vi "ConfMappOut.vi"(8 "error in (no error)":errorcluster, 11 "ConfMapOut In":string[](array[string])) -> (0 "error out":errorcluster, 1 "Discard?":bool, 3 "ConfMapOut Out":string[](array[string]))   [LabVIEW 2014]
uses:
  TypeDefs/LogicParsedExpression.ctl
  SeqLoop.lvlib
panel:
  in  "Formula":string
  in  "Tipo de Salida":string(combo)
  in  "Stop Med":bool
  in  "Add Med":bool
  in  "Descripción":string
  in  "Nro.":i32
  in  "Nro. Hardware":i32
  in  "Bit":i32
  in  "Habilitada":bool
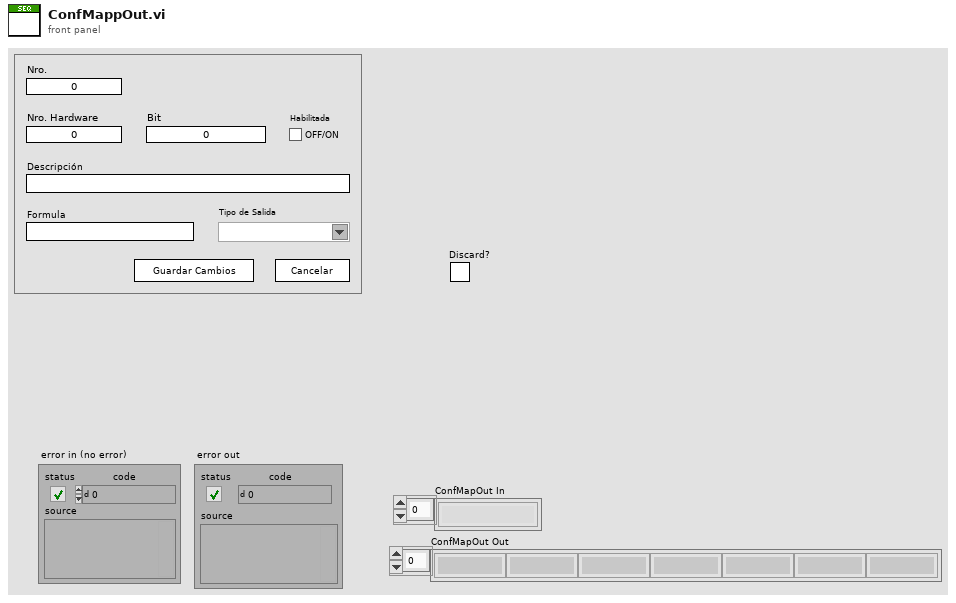
[diagram p1: front panel]
types:
  T1 = typedef "SeqLoop.lvlib/LogicParsedExpression.ctl" = cluster{"RPN ":string[], "Variables":string[], "Ctes":string[], "Formula":string, "Message":string}
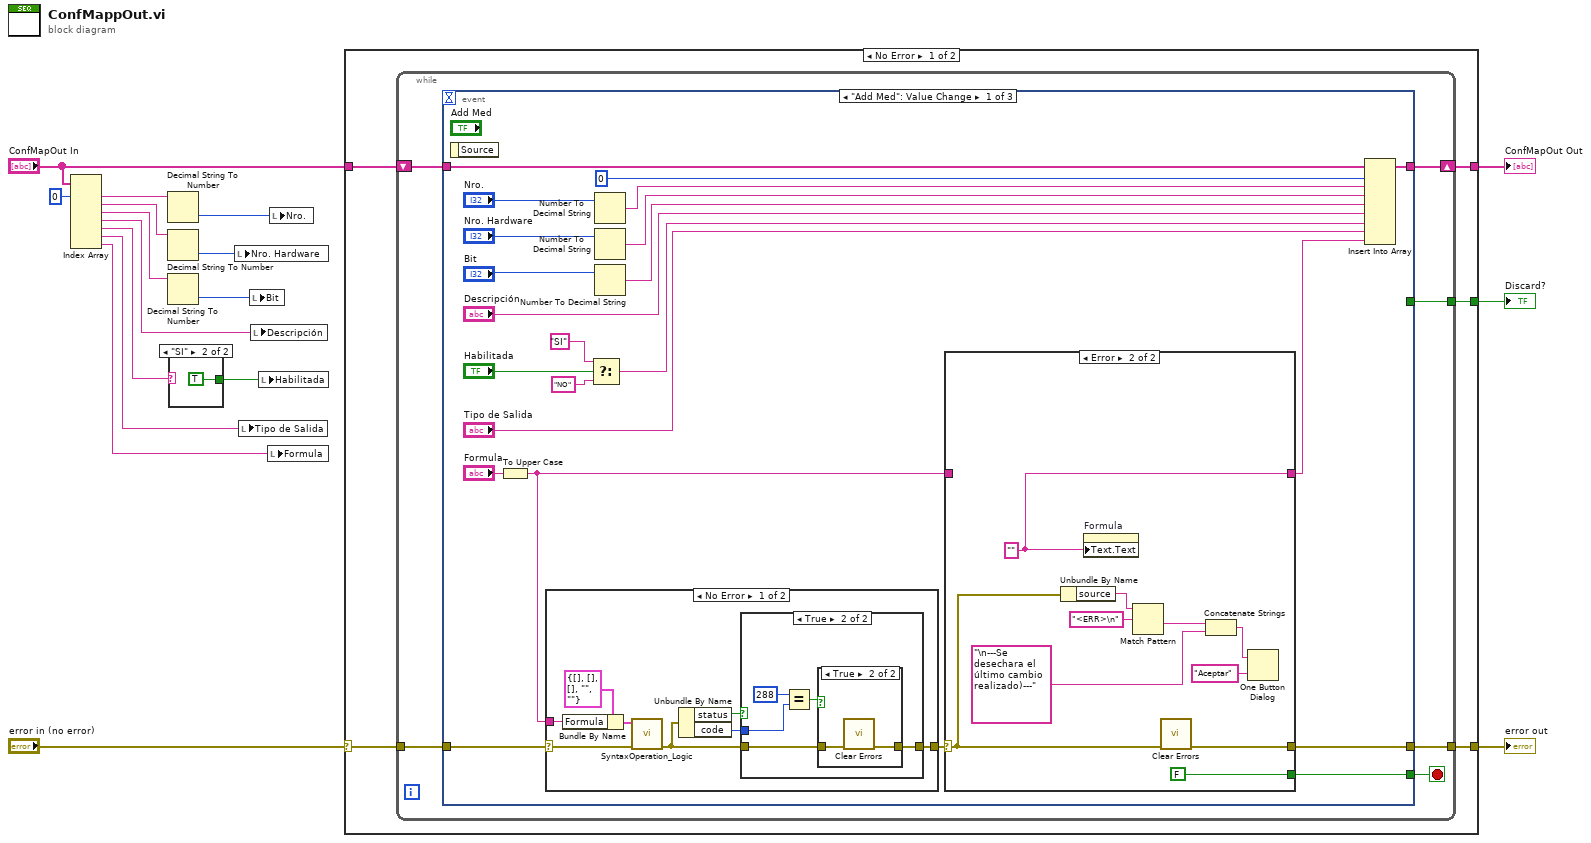
[diagram p0: block diagram]
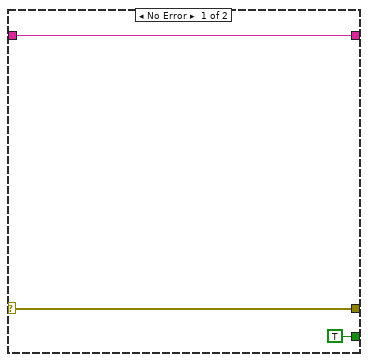
[diagram p6: hidden frame]
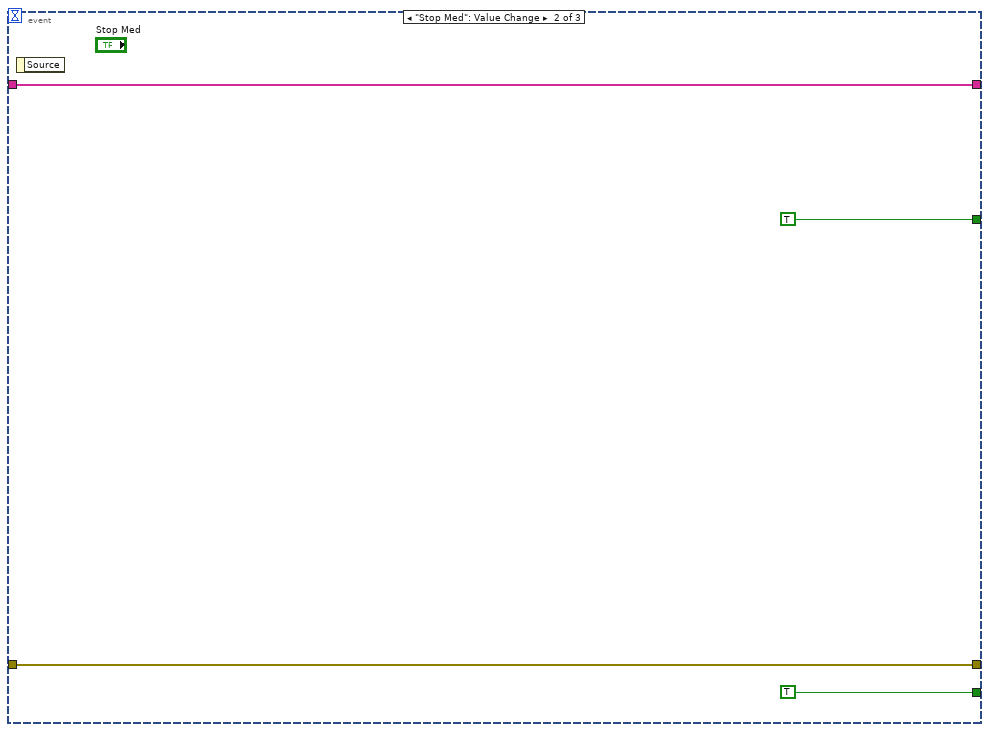
[diagram p7: hidden frame]
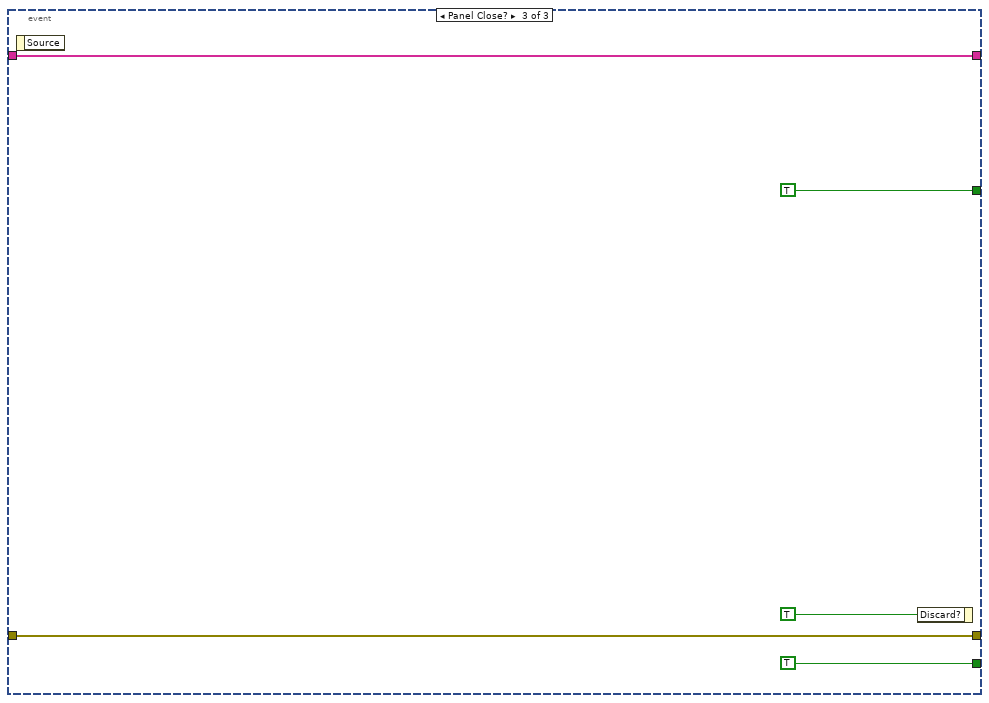
[diagram p8: hidden frame]
diagram:
  n1 = Index Array(array="ConfMapOut In", index #1=0 ("index")) -> (element #1=w12:string, element #2=w7:string, element #3=w6:string, element #4=w8:string, element #5=w5:string, element #6=w2:string, element #7=w1:string)  [unwired: 6 in]
  n2 = Decimal String To Number(string=w12) -> (number=w11:i32)  [unwired: 2 in, 1 out]
  n3 = Decimal String To Number(string=w7) -> (number=w10:i32)  [unwired: 2 in, 1 out]
  n4 = Decimal String To Number(string=w6) -> (number=w9:i32)  [unwired: 2 in, 1 out]
  n5 = case shown="\"SI\"" w5 {
    tunnel: [_ TRUE] -> w4
    frame "NO", Default {
    }
    frame "SI" {
    }
  }
  n6 = local write "Nro. Hardware"(w10) -> ()
  n7 = local write "Tipo de Salida"(w2) -> ()
  n8 = local write "Bit"(w9) -> ()
  n9 = local write "Descripción"(w8) -> ()
  n10 = local write "Habilitada"(w4) -> ()
  n11 = local write "Formula"(w1) -> ()
  n12 = local write "Nro."(w11) -> ()
  n13 = case shown="No Error" "error in (no error)" {
    selector: "error in (no error)" -> [w21 w93]
    tunnel: [w23 w93] -> w16
    tunnel: "ConfMapOut In" -> [w20 w92]
    tunnel: [w22 w92] -> w15
    tunnel: [w19 _] -> w3
    frame No Error {
      n14 = while {
        tunnel: w21 -> [w28]
        tunnel: [w29] -> w23
        shift-right: [w24] -> w22
        shift-left: w20 -> [w26]
        tunnel: [w25] -> w19
        stop <- w27 stop-if-true
        n15 = event shown="[0] \"Add Med\": Value Change" {
          selector: _ -> [_ _ _]
          dyn-events: _ -> [_ _ _]
          timeout: _ -> [_ _ _]
          tunnel: [w34 w85 w88] -> w29
          tunnel: w28 -> [w35 w85 w88]
          tunnel: [w33 TRUE ("Discard?") TRUE ("Discard?")] -> w27
          tunnel: w26 -> [w39 w84 w89]
          tunnel: [w45 w84 w89] -> w24
          tunnel: [_ TRUE ("Discard?") TRUE ("Discard?")] -> w25
          event "Add Med": Value Change {
            n16 = event-data() -> ()  [unwired: 1 in, 1 out]
            n17 = To Upper Case(1:"Formula") -> (0:w30:string)
            n18 = case shown="No Error" w35 {
              selector: w35 -> [w53 w69]
              tunnel: w30 -> [w57 _]
              tunnel: [w55 w69] -> w36
              frame No Error {
                n19 = Bundle By Name(cluster=T1 {"RPN "=[], "Variables"=[], "Ctes"=[], "Formula"="", "Message"=""} ("Logical Parsed Expression"), "Formula"=w57) -> (w58:T1)
                n20 = call "SyntaxOperation_Logic.vi"("error in (no error)"=w53, "Logical Parsed Expression"=w58) -> ("error out"=w54:errorcluster)  [unwired: 6 in, 3 out]
                n21 = Unbundle By Name(w54) -> ("status"=w56:bool, "code"=w52:i32)
                n22 = case shown="True" w56 {
                  tunnel: [w60 w61] -> w55
                  tunnel: w54 -> [w60 w62]
                  tunnel: w52 -> [_ w65]
                  frame False {
                  }
                  frame True {
                    n23 = Equal?(x=288, y=w65) -> (x = y?=w63:bool)
                    n24 = case shown="True" w63 {
                      tunnel: w62 -> [w66 w68]
                      tunnel: [w66 w67] -> w61
                      frame False {
                      }
                      frame True {
                        n25 = call <vilib>:"Clear Errors.vi"("error in (no error)"=w68) -> ("error out"=w67:errorcluster)  [unwired: 5 in, 1 out]
                      }
                    }
                  }
                }
              }
              frame Error {
              }
            }
            n26 = Select(t="SI" ("Descripción 2"), s="Habilitada", f="NO" ("Descripción 2")) -> (s? t:f=w40:string)
            n27 = Number To Decimal String(number="Nro.") -> (decimal integer string=w44:string)  [unwired: 1 in]
            n28 = Number To Decimal String(number="Nro. Hardware") -> (decimal integer string=w43:string)  [unwired: 1 in]
            n29 = Number To Decimal String(number="Bit") -> (decimal integer string=w42:string)  [unwired: 1 in]
            n30 = case shown="Error" w36 {
              selector: w36 -> [w71 w78]
              tunnel: [w71 w77] -> w34
              tunnel: [TRUE ("Discard?") FALSE ("Discard?")] -> w33
              tunnel: [w70 w73] -> w32
              tunnel: w30 -> [w70 _]
              frame No Error {
              }
              frame Error {
                w73 = "" ("Text.Text")
                n31 = Unbundle By Name(w78) -> ("source"=w80:string)
                n32 = property on="Formula" class="Str"("Text.Text"=w73) -> ()  [unwired: 2 in, 2 out]
                n33 = Match Pattern(string=w80, regular expression="<ERR>\n") -> (after substring=w74:string)  [unwired: 1 in, 3 out]
                n34 = call <vilib>:"Clear Errors.vi"("error in (no error)"=w78) -> ("error out"=w77:errorcluster)  [unwired: 5 in, 1 out]
                n35 = Concatenate Strings(w74, "\n---Se desechara el último cambio realizado)---" ("button name (\"OK\")")) -> (w82:string)
                n36 = One Button Dialog(message=w82, button name ("OK")="Aceptar") -> ()  [unwired: 1 out]
              }
            }
            n37 = Insert Into Array(array=w39, index=0, new element #1=w44, new element #2=w43, new element #3=w42, new element #4="Descripción", new element #5=w40, new element #6="Tipo de Salida", new element #7=w32) -> (w45:string[])
          }
          event "Stop Med": Value Change {
            n38 = event-data() -> ()  [unwired: 1 in, 1 out]
          }
          event Panel Close? {
            n39 = event-data() -> ()  [unwired: 1 in, 1 out]
            n40 = event-data("Discard?"=TRUE) -> ()  [unwired: 1 in, 1 out]
          }
        }
      }
    }
    frame Error {
    }
  }
  "error out" <- w16
  "ConfMapOut Out" <- w15
  "Discard?" <- w3
